vi "XML setApiRequest.vi"(11 "PIM API Request":T1={"#attributes"={"xmlns"="http://www.summitekinstruments.com", "xmlns:xsi"="http://www.w3.org/2001/XMLSchema-instance", "xsi:schemaLocation"="http://www.summitekinstruments.com PIMXMLSchema.xsd"}, "Commands"={"#attributes"={"Token"="", "Legacy"=FALSE}, "Command"=[]}}) -> (3 "Formatted XML":string, 5 "Time to Translate":u32)   [LabVIEW 2011]
uses:
  Controls/PIM.API.REQUEST.ctl
  Controls/PIM.API.Command.Collection.ctl
  Controls/PIM.API.Command.Unique.ctl
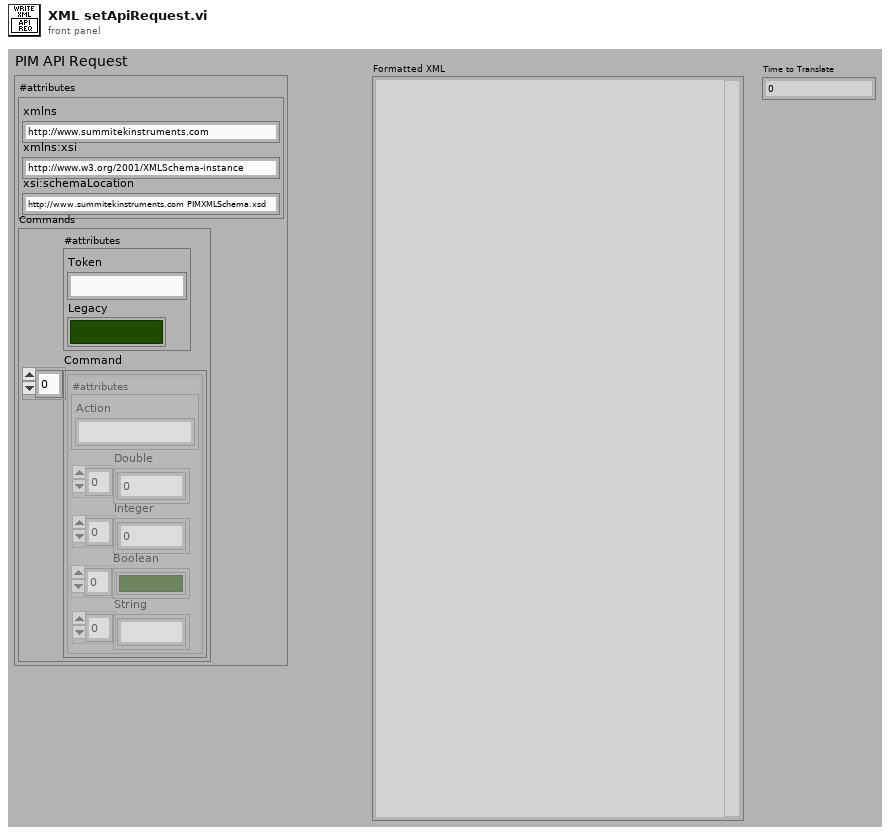
[diagram p1: front panel]
types:
  T1 = typedef "PIM.API.REQUEST.ctl" = cluster{"#attributes":cluster{"xmlns":string, "xmlns:xsi":string, "xsi:schemaLocation":string}, "Commands":T2}
  T2 = typedef "PIM.API.Command.Collection.ctl" = cluster{"#attributes":cluster{"Token":string, "Legacy":bool}, "Command":T3[]}
  T3 = typedef "PIM.API.Command.Unique.ctl" = cluster{"#attributes":cluster{"Action":string}, "Double":dbl[], "Integer":i32[], "Boolean":bool[], "String":string[]}
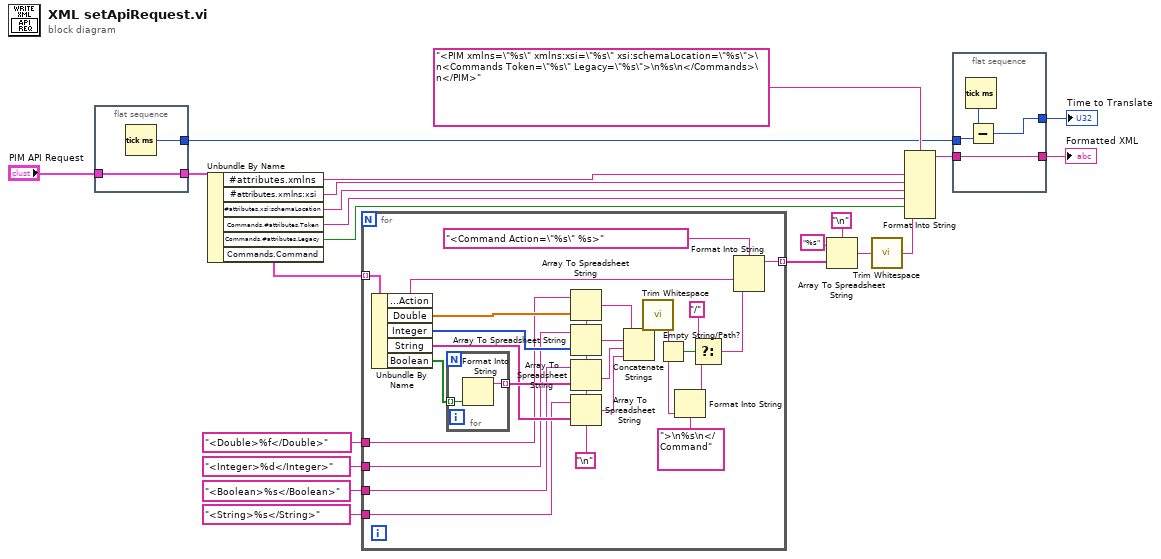
[diagram p0: block diagram]
diagram:
  n1 = flat-sequence {
    tunnel: "PIM API Request" -> [w24]
    tunnel: [w24] -> w7
    tunnel: [w23] -> w4
    frame #0 {
      n2 = Tick Count (ms)() -> (millisecond timer value=w23:u32)
    }
  }
  n3 = Unbundle By Name(w7) -> ("#attributes.xmlns"=w21:string, "#attributes.xmlns:xsi"=w20:string, "#attributes.xsi:schemaLocation"=w19:string, "Commands.#attributes.Token"=w1:string, "Commands.#attributes.Legacy"=w18:bool, "Commands.Command"=w17:T3[])
  n4 = for {
    tunnel: w17 -> [w49] mode=indexing
    tunnel: "<Double>%f</Double>" -> [w41]
    tunnel: "<Integer>%d</Integer>" -> [w40]
    tunnel: "<Boolean>%s</Boolean>" -> [w39]
    tunnel: "<String>%s</String>" -> [w38]
    tunnel: [w31] -> w12 mode=indexing
    w37 = "\n" ("delimiter (Tab)")
    n5 = Unbundle By Name(w49) -> ("#attributes.Action"=w47:string, "Double"=w42:dbl[], "Integer"=w43:i32[], "String"=w44:string[], "Boolean"=w46:bool[])
    n6 = for {
      tunnel: w46 -> [w51] mode=indexing
      tunnel: [w50] -> w45 mode=indexing
      n7 = Format Into String(w51) -> (resulting string=w50:string)  [unwired: 3 in, 1 out]
    }
    n8 = Array To Spreadsheet String(delimiter (Tab)=w37, array=w42, 3:w41) -> (spreadsheet string=w35:string)
    n9 = Array To Spreadsheet String(delimiter (Tab)=w37, array=w43, 3:w40) -> (spreadsheet string=w34:string)
    n10 = Array To Spreadsheet String(delimiter (Tab)=w37, array=w45, 3:w39) -> (spreadsheet string=w33:string)
    n11 = Array To Spreadsheet String(delimiter (Tab)=w37, array=w44, 3:w38) -> (spreadsheet string=w32:string)
    n12 = Concatenate Strings(w35, w34, w33, w32) -> (w36:string)
    n13 = call <vilib>:"Trim Whitespace.vi"("string"=w36) -> ("trimmed string"=w29:string)  [unwired: 1 in]
    n14 = Empty String/Path?(string/path=w29) -> (empty?=w30:bool)
    n15 = Format Into String(format string=">\n%s\n</Command", w29) -> (resulting string=w26:string)  [unwired: 2 in, 1 out]
    n16 = Select(t="/", s=w30, f=w26) -> (s? t:f=w25:string)
    n17 = Format Into String(format string="<Command Action=\"%s\" %s>", w47, w25) -> (resulting string=w31:string)  [unwired: 2 in, 1 out]
  }
  n18 = Array To Spreadsheet String(delimiter (Tab)="\n", array=w12, 3:"%s" ("initial string")) -> (spreadsheet string=w10:string)
  n19 = call <vilib>:"Trim Whitespace.vi"("string"=w10) -> ("trimmed string"=w2:string)  [unwired: 1 in]
  n20 = Format Into String(format string="<PIM xmlns=\"%s\" xmlns:xsi=\"%s\" xsi:schemaLocation=\"%s\">\n<Commands Token=\"%s\" Legacy=\"%s\">\n%s\n</Commands>\n</PIM>", w21, w20, w19, w1, w18, w2) -> (resulting string=w6:string)  [unwired: 2 in, 1 out]
  n21 = flat-sequence {
    tunnel: w6 -> [w55]
    tunnel: [w55] -> w5
    tunnel: w4 -> [w54]
    tunnel: [w52] -> w3
    frame #0 {
      n22 = Tick Count (ms)() -> (millisecond timer value=w53:u32)
      n23 = Subtract(x=w53, y=w54) -> (x-y=w52:u32)
    }
  }
  "Formatted XML" <- w5
  "Time to Translate" <- w3
